vi "TDC_修正后数据处理.vi"() -> ()   [LabVIEW 2014]
uses:
  <vilib>/Utility/file.llb/Read From Spreadsheet File (DBL).vi
panel:
  out "分布谱":dbl[](graph)
  out "b细计数":dbl[](array[numeric]) caption="第一行" format="%0.3f"
  in  "b细计数文件":path caption="b"
  out "a细计数":dbl[](array[numeric]) caption="第一行" format="%0.3f"
  in  "a细计数文件":path caption="a"
  out "粗计数":dbl[](array[numeric]) caption="第一行" format="%0.3f"
  in  "粗计数文件":path caption="粗"
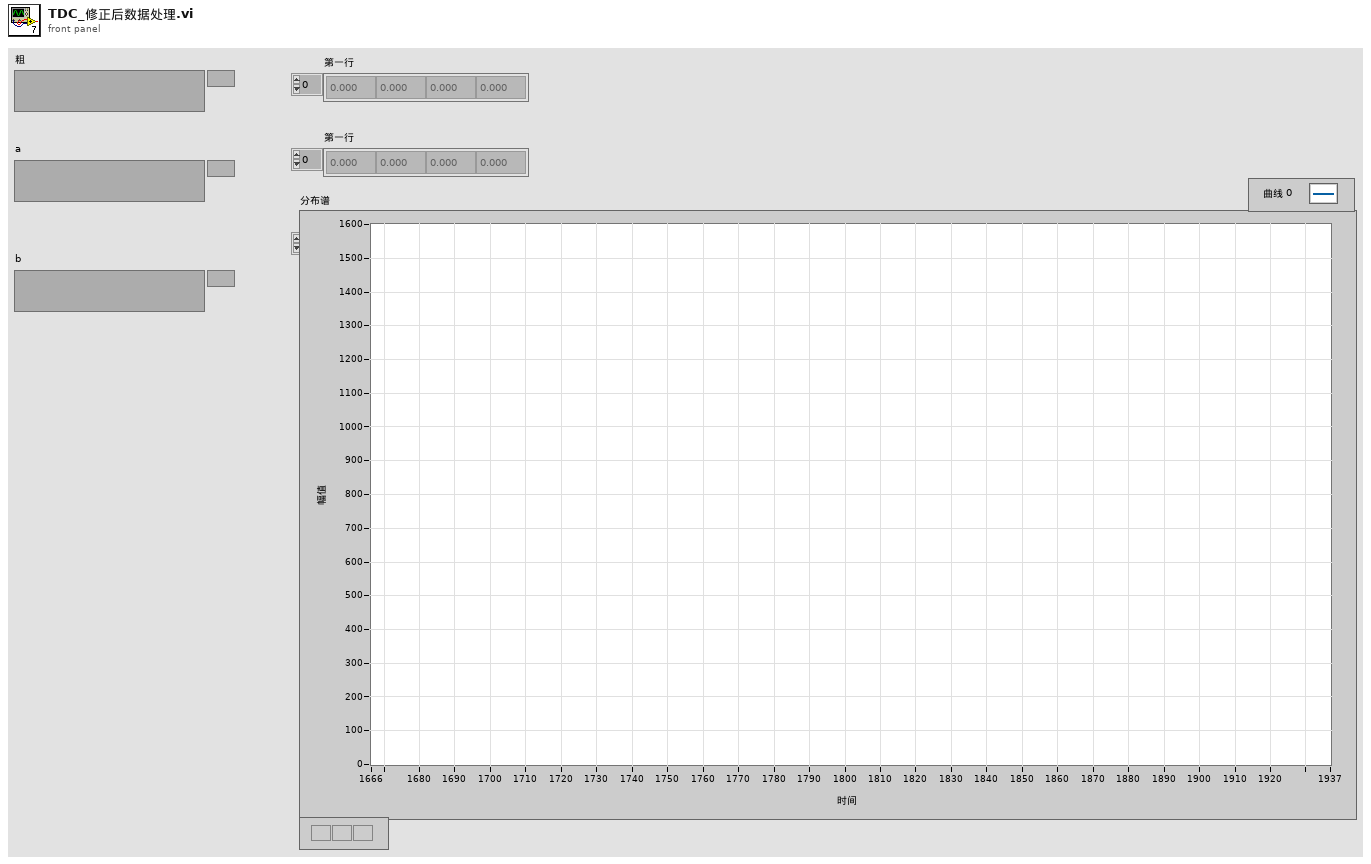
[diagram p1: front panel]
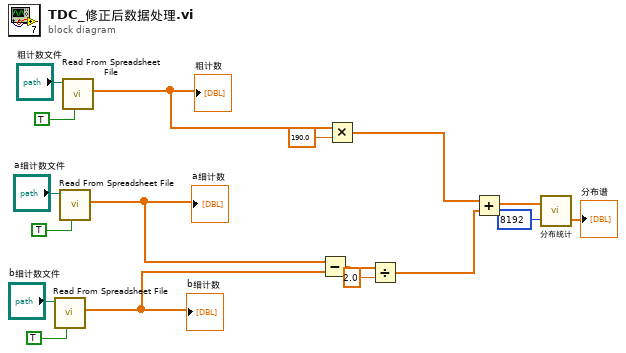
[diagram p0: block diagram]
diagram:
  n1 = call-poly <vilib>:"Read From Spreadsheet File.vi"("transpose (no:F)"=TRUE, "file path (dialog if empty)"="b细计数文件") -> ("first row"=w10:dbl[])  [unwired: 5 in, 4 out]
  "b细计数" <- w10
  n2 = call-poly <vilib>:"Read From Spreadsheet File.vi"("transpose (no:F)"=TRUE, "file path (dialog if empty)"="a细计数文件") -> ("first row"=w11:dbl[])  [unwired: 5 in, 4 out]
  "a细计数" <- w11
  n3 = call-poly <vilib>:"Read From Spreadsheet File.vi"("transpose (no:F)"=TRUE, "file path (dialog if empty)"="粗计数文件") -> ("first row"=w6:dbl[])  [unwired: 5 in, 4 out]
  "粗计数" <- w6
  n4 = Subtract(x=w11, y=w10) -> (x-y=w8:dbl[])
  n5 = Multiply(x=w6, y=190.0) -> (x*y=w5:dbl[])
  n6 = Divide(x=w8, y=2.0) -> (x/y=w4:dbl[])
  n7 = Add(x=w5, y=w4) -> (x+y=w3:dbl[])
  n8 = call "分布统计.vi"("道数"=8192, "数组"=w3) -> ("分布谱"=→"分布谱":dbl[])  [unwired: 1 out]
